vi "test_TCP_2_parseRead_p1.vi"(7 "input_stringNew":string, 8 "input_index":u16, 9 "input_arrayIndices":u16[](array[numeric]), 10 "input_haveStart":bool, 11 "input_stringAccum":string) -> (0 "output_index":u16, 1 "output_arrayIndices":u16[](array[numeric]), 2 "output_haveStart":bool, 3 "output_stringAccum":string, 5 "output_haveCmd":bool)   [LabVIEW 2014]
panel:
  out "length":i32
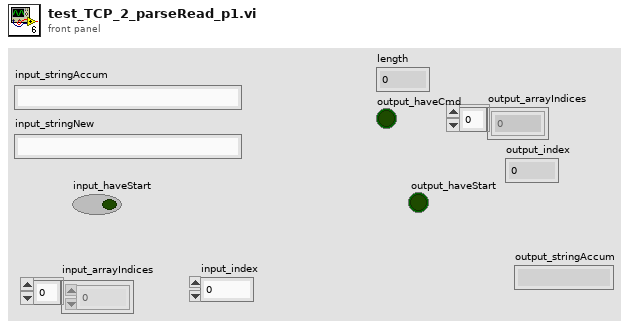
[diagram p1: front panel]
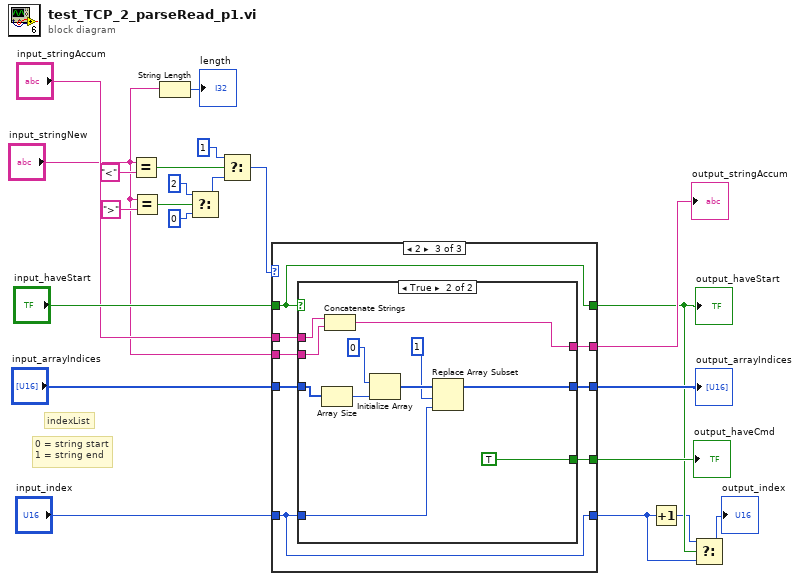
[diagram p0: block diagram]
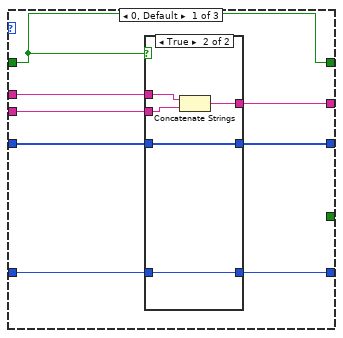
[diagram p2: hidden frame]
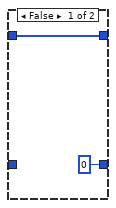
[diagram p3: hidden frame]
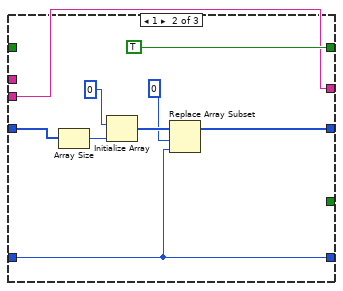
[diagram p4: hidden frame]
diagram:
  # "0 = string start\n1 = string end"
  # "indexList"
  n1 = Equal?(x="input_stringNew", y="<") -> (x = y?=w17:bool)
  n2 = Equal?(x="input_stringNew", y=">") -> (x = y?=w14:bool)
  n3 = String Length(string="input_stringNew") -> (length=→"length":i32)
  n4 = Select(t=u16 2, s=w14, f=u16 0) -> (s? t:f=w13:u16)
  n5 = Select(t=u16 1, s=w17, f=w13) -> (s? t:f=w15:u16)
  n6 = case shown="2" w15 {
    tunnel: [w30 TRUE w51] -> w6
    tunnel: "input_arrayIndices" -> [w26 w46 w54]
    tunnel: [w25 w42 w53] -> w19
    tunnel: "input_haveStart" -> [w30 _ w51]
    tunnel: "input_index" -> [w24 w39 w52]
    tunnel: [w23 w39 w52] -> w4
    tunnel: "input_stringNew" -> [w29 w38 w49]
    tunnel: "input_stringAccum" -> [w28 _ w50]
    tunnel: [w27 w38 w48] -> w8
    tunnel: [_ _ w47] -> w7
    frame 0, Default {
      n7 = case shown="True" w30 {
        tunnel: w29 -> [_ w36]
        tunnel: w28 -> [_ w37]
        tunnel: [_ w35] -> w27
        tunnel: w26 -> [w32 w34]
        tunnel: [w32 w34] -> w25
        tunnel: [u16 0 ("input_index") w33] -> w23
        tunnel: w24 -> [_ w33]
        frame False {
        }
        frame True {
          n8 = Concatenate Strings(w37, w36) -> (w35:string)
        }
      }
    }
    frame 1 {
      n9 = Array Size(array=w46) -> (size(s)=w45:i32)
      n10 = Initialize Array(u16 0, w45) -> (w43:u16[])
      n11 = Replace Array Subset(array=w43, new element=w39, index=0) -> (w42:u16[])
    }
    frame 2 {
      n12 = case shown="True" w51 {
        tunnel: w54 -> [w55 w66]
        tunnel: [w55 w62] -> w53
        tunnel: w52 -> [_ w60]
        tunnel: w50 -> [_ w59]
        tunnel: w49 -> [_ w58]
        tunnel: [_ w57] -> w48
        tunnel: [_ TRUE] -> w47
        frame False {
          # "do nothing"
        }
        frame True {
          n13 = Array Size(array=w66) -> (size(s)=w65:i32)
          n14 = Concatenate Strings(w59, w58) -> (w57:string)
          n15 = Initialize Array(u16 0, w65) -> (w63:u16[])
          n16 = Replace Array Subset(array=w63, new element=w60, index=1) -> (w62:u16[])
        }
      }
    }
  }
  "output_stringAccum" <- w8
  "output_haveStart" <- w6
  "output_arrayIndices" <- w19
  "output_haveCmd" <- w7
  n17 = Increment(x=w4) -> (x+1=w5:u16)
  n18 = Select(t=w5, s=w6, f=w4) -> (s? t:f=→"output_index":u16)
